vi "niECAT_EnumPDOs.vi"   [LabVIEW 2020]
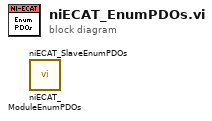
[diagram p0: block diagram]
diagram:
  n1 = call <vilib>:"niECAT_ModuleEnumPDOs.vi"() -> ()  [unwired: 8 in, 4 out]
  n2 = call <vilib>:"niECAT_SlaveEnumPDOs.vi"() -> ()  [unwired: 8 in, 4 out]
